vi "Create Item Paths.vi"(5 "Folder Row":string, 7 "Type Row":string, 10 "Folder Tree":T1[](array[typedef]), 11 "Type Tree":T3[](array[typedef])) -> (2 "Project Path":string, 3 "Type Path":string)   [LabVIEW 2018, in "LVClassByRef.lvlib"]
uses:
  <resource>/Framework/Providers/LVClassByRef/LVClassByRef.lvlib
  <resource>/Framework/Providers/LVClassByRef/Type Item.ctl
  <resource>/Framework/Providers/LVClassByRef/Tree Item.ctl
  <vilib>/Utility/Data Type/Type Definitions/Data Type.ctl
  <resource>/Framework/Providers/LVClassByRef/Folder Item.ctl
  <vilib>/Utility/Data Type/NI_Data Type.lvlib
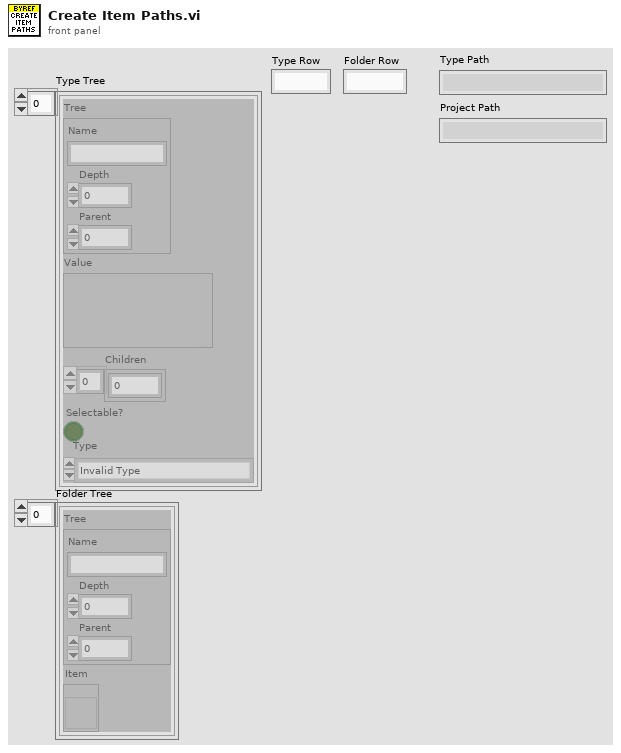
[diagram p1: front panel]
types:
  T1 = typedef "LVClassByRef.lvlib/Folder Item.ctl" = cluster{"Tree":T2, "Item":refnum<vi>}
  T2 = typedef "LVClassByRef.lvlib/Tree Item.ctl" = cluster{"Name":string, "Depth":i32, "Parent":i32}
  T3 = typedef "LVClassByRef.lvlib/Type Item.ctl" = cluster{"Tree":T2, "Value":variant, "Children":i32[], "Selectable?":bool, "Type":T4}
  T4 = typedef "NI_Data Type.lvlib/Data Type.ctl" = enum8{"Invalid Type", "Void", "I8", "I16", "I32", "I64", "U8", "U16", "U32", "U64", "Single Float", "Double Float", "Extended Float", "Single Complex", "Double Complex", "Extended Complex", "Enum U8", "Enum U16", "Enum U32", "Enum U64", "Single Float With Unit", "Double Float With Unit", "Extended Float With Unit", "Single Complex with Unit", "Double Complex with Unit", "Extended Complex with Unit", "Boolean", "String", "Path", "Picture", "Tag", "Array", "Cluster", "Variant", "LV Variant", "Waveform", "Timestamp", "Digital Waveform", "Digital Data", "ExpressData", "Refnum", "External Data", "VI", "Poly VI", "LabVIEW Class Instance", "Fixed Point"}
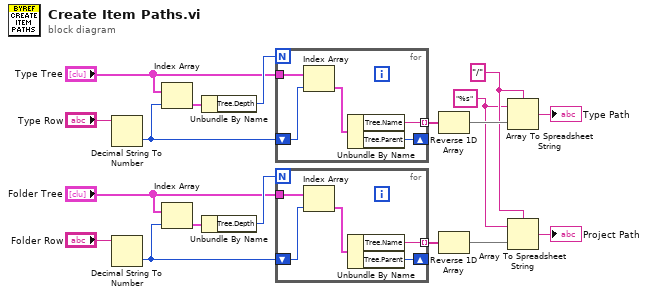
[diagram p0: block diagram]
diagram:
  w7 = "/" ("delimiter (Tab)")
  w6 = "%s" ("format string")
  n1 = Decimal String To Number(string="Type Row") -> (number=w2:i32)  [unwired: 2 in, 1 out]
  n2 = Decimal String To Number(string="Folder Row") -> (number=w3:i32)  [unwired: 2 in, 1 out]
  n3 = Index Array(array="Type Tree", index=w2) -> (element=w18:T3)
  n4 = Index Array(array="Folder Tree", index=w3) -> (element=w10:T1)
  n5 = Unbundle By Name(w18) -> ("Tree.Depth"=w17:i32)
  n6 = Unbundle By Name(w10) -> ("Tree.Depth"=w11:i32)
  n7 = for {
    N: w17 -> [_]
    tunnel: "Type Tree" -> [w23]
    shift-right: [w20] -> _
    shift-left: w2 -> [w22]
    tunnel: [w19] -> w15 mode=indexing
    n8 = Index Array(array=w23, index=w22) -> (element=w21:T3)
    n9 = Unbundle By Name(w21) -> ("Tree.Name"=w19:string, "Tree.Parent"=w20:i32)
  }
  n10 = for {
    N: w11 -> [_]
    tunnel: "Folder Tree" -> [w28]
    shift-right: [w25] -> _
    shift-left: w3 -> [w27]
    tunnel: [w24] -> w12 mode=indexing
    n11 = Index Array(array=w28, index=w27) -> (element=w26:T1)
    n12 = Unbundle By Name(w26) -> ("Tree.Name"=w24:string, "Tree.Parent"=w25:i32)
  }
  n13 = Reverse 1D Array(array=w15) -> (reversed array=w14:string[])
  n14 = Reverse 1D Array(array=w12) -> (reversed array=w13:string[])
  n15 = Array To Spreadsheet String(delimiter (Tab)=w7, array=w14, 3:w6) -> (spreadsheet string=→"Type Path":string)
  n16 = Array To Spreadsheet String(delimiter (Tab)=w7, array=w13, 3:w6) -> (spreadsheet string=→"Project Path":string)
